vi "Main5.vi"(4 "מק\"ט המכלל":string, 5 "מספר סידורי":string, 7 "מפעיל":string="ANS", 8 "error":errorcluster, 11 "Path for Log":path) -> (0 "error IO":errorcluster)   [LabVIEW 2014]
uses:
  StopForLog.vi
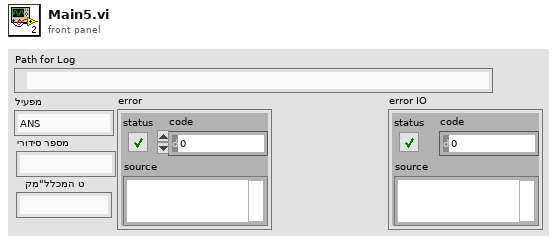
[diagram p1: front panel]
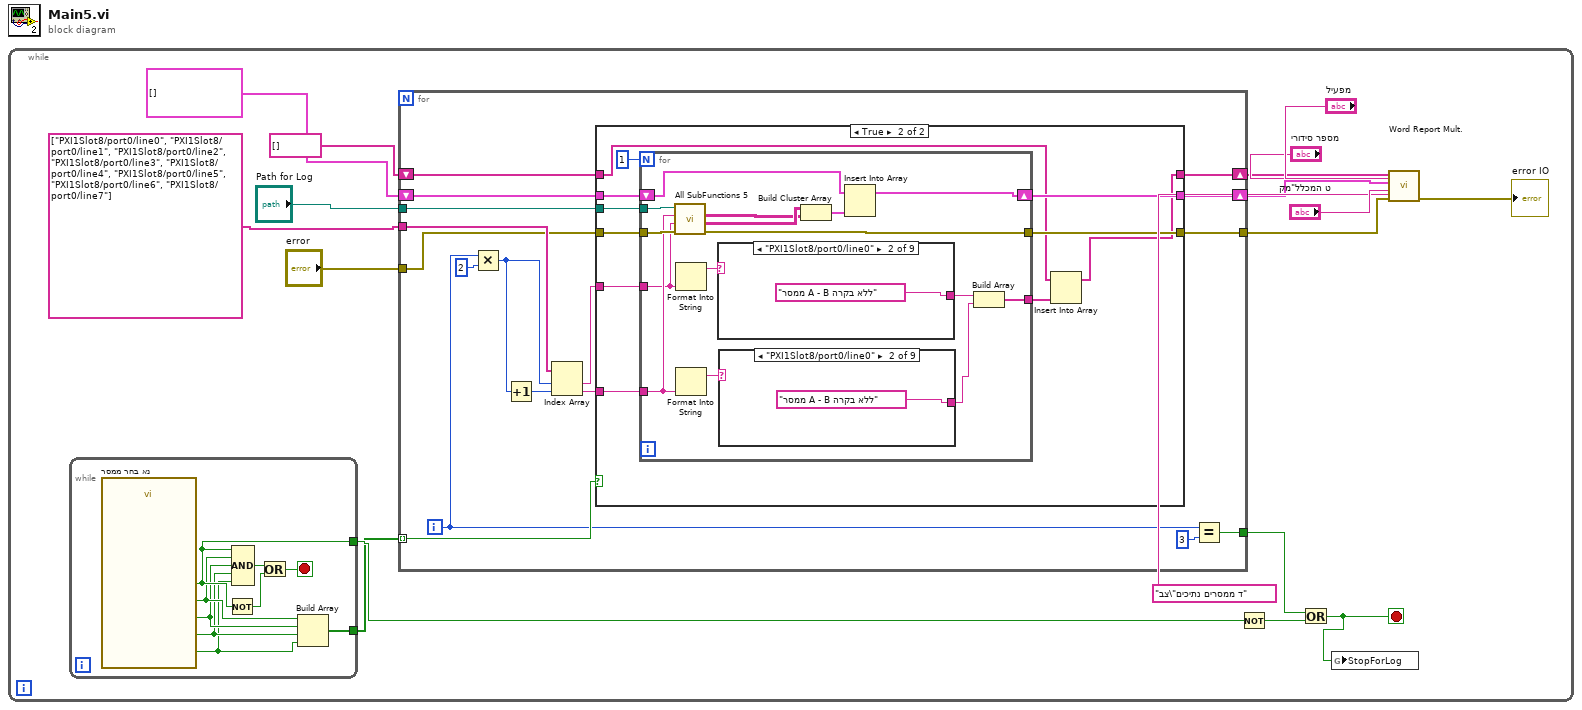
[diagram p0: block diagram]
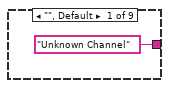
[diagram p3: hidden frame]
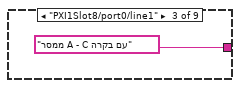
[diagram p4: hidden frame]
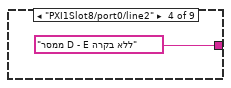
[diagram p5: hidden frame]
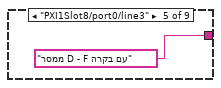
[diagram p6: hidden frame]
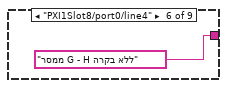
[diagram p7: hidden frame]
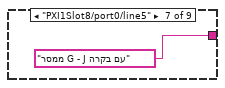
[diagram p8: hidden frame]
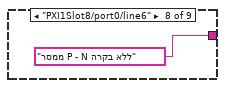
[diagram p9: hidden frame]
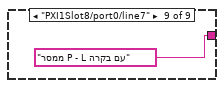
[diagram p10: hidden frame]
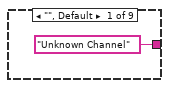
[diagram p11: hidden frame]
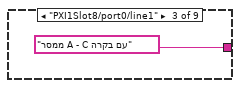
[diagram p12: hidden frame]
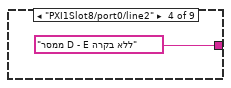
[diagram p13: hidden frame]
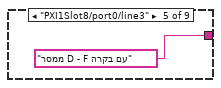
[diagram p14: hidden frame]
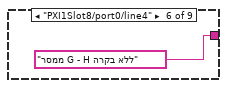
[diagram p15: hidden frame]
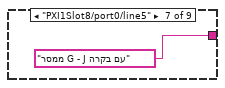
[diagram p16: hidden frame]
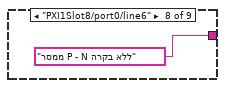
[diagram p17: hidden frame]
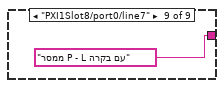
[diagram p18: hidden frame]
diagram:
  n1 = while {
    stop <- w1 stop-if-true
    n2 = while {
      tunnel: [w25] -> w18
      tunnel: [w26] -> w17
      stop <- w19 stop-if-true
      n3 = call "נא בחר ממסר.vi"() -> ("P - N/L"=w21:bool, "G - H/J"=w22:bool, "D - E/F"=w23:bool, "A - B/C"=w24:bool, "OK"=w25:bool)  [unwired: 13 in, 2 out]
      n4 = Not(x=w25) -> (.not. x?=w27:bool)
      n5 = Compound Arithmetic op=AND(w25, w24, w23, w22, w21) -> (w20:bool)
      n6 = Or(x=w20, y=w27) -> (x .or. y?=w19:bool)
      n7 = Build Array(w24, w23, w22, w21) -> (w26:bool[])
    }
    n8 = for {
      tunnel: w17 -> [w44] mode=indexing
      tunnel: tag[] ["PXI1Slot8/port0/line0", "PXI1Slot8/port0/line1", "PXI1Slot8/port0/line2", "PXI1Slot8/port0/line3", "PXI1Slot8/port0/line4", "PXI1Slot8/port0/line5", "PXI1Slot8/port0/line6", "PXI1Slot8/port0/line7"] -> [w43]
      tunnel: "Path for Log" -> [w37]
      tunnel: [w36] -> w6
      tunnel: "error" -> [w35]
      shift-right: [w33] -> w8
      shift-left: cluster{"appended array":string[][]}[] [] ("array of clusters") -> [w34]
      shift-right: [w31] -> w4
      shift-left: string[] [] ("Array 2") -> [w32]
      tunnel: [w28] -> w2
      i -> [w30]
      n9 = Multiply(x=w30, y=2) -> (x*y=w41:i32)
      n10 = Increment(x=w41) -> (x+1=w40:i32)
      n11 = Index Array(array=w43, index #1=w41, index #2=w40) -> (element #1=w39:tag, element #2=w38:tag)
      n12 = case shown="True" w44 {
        tunnel: w39 -> [_ w51]
        tunnel: w38 -> [_ w50]
        tunnel: w37 -> [_ w58]
        tunnel: [w47 w57] -> w36
        tunnel: w35 -> [w47 w56]
        tunnel: w34 -> [w46 w55]
        tunnel: [w46 w54] -> w33
        tunnel: w32 -> [w45 w53]
        tunnel: [w45 w52] -> w31
        frame False {
        }
        frame True {
          n13 = for {
            N: 1 -> [_]
            tunnel: w58 -> [w73]
            tunnel: [w72] -> w57
            tunnel: w56 -> [w71]
            shift-right: [w67] -> w54
            shift-left: w55 -> [w69]
            tunnel: w51 -> [w64]
            tunnel: w50 -> [w65]
            tunnel: [w66] -> w49
            n14 = call "All SubFunctions 5.vi"("error"=w71, "lines 1"=w64, "lines"=w65, "Path for Log"=w73) -> ("error IO"=w72:errorcluster, "appended array 1"=w62:string[][], "appended array"=w61:string[][])  [unwired: 5 in]
            n15 = Format Into String(w64) -> (resulting string=w70:string)  [unwired: 3 in, 1 out]
            n16 = Format Into String(w65) -> (resulting string=w59:string)  [unwired: 3 in, 1 out]
            n17 = case shown="\"PXI1Slot8/port0/line0\"" w70 {
              tunnel: ["Unknown Channel" "ממסר A - B ללא בקרה" "ממסר A - C עם בקרה" "ממסר D - E ללא בקרה" "ממסר D - F עם בקרה" "ממסר G - H ללא בקרה" "ממסר G - J עם בקרה" "ממסר P - N ללא בקרה" "ממסר P - L עם בקרה"] -> w63
              frame "", Default {
              }
              frame "PXI1Slot8/port0/line0" {
              }
              frame "PXI1Slot8/port0/line1" {
              }
              frame "PXI1Slot8/port0/line2" {
              }
              frame "PXI1Slot8/port0/line3" {
              }
              frame "PXI1Slot8/port0/line4" {
              }
              frame "PXI1Slot8/port0/line5" {
              }
              frame "PXI1Slot8/port0/line6" {
              }
              frame "PXI1Slot8/port0/line7" {
              }
            }
            n18 = case shown="\"PXI1Slot8/port0/line0\"" w59 {
              tunnel: ["Unknown Channel" "ממסר A - B ללא בקרה" "ממסר A - C עם בקרה" "ממסר D - E ללא בקרה" "ממסר D - F עם בקרה" "ממסר G - H ללא בקרה" "ממסר G - J עם בקרה" "ממסר P - N ללא בקרה" "ממסר P - L עם בקרה"] -> w60
              frame "", Default {
              }
              frame "PXI1Slot8/port0/line0" {
              }
              frame "PXI1Slot8/port0/line1" {
              }
              frame "PXI1Slot8/port0/line2" {
              }
              frame "PXI1Slot8/port0/line3" {
              }
              frame "PXI1Slot8/port0/line4" {
              }
              frame "PXI1Slot8/port0/line5" {
              }
              frame "PXI1Slot8/port0/line6" {
              }
              frame "PXI1Slot8/port0/line7" {
              }
            }
            n19 = Build Cluster Array(w62, w61) -> (w68:cluster{"appended array":string[][]}[])
            n20 = Insert Into Array(array=w69, new element=w68) -> (w67:cluster{"appended array":string[][]}[])  [unwired: 1 in]
            n21 = Build Array(w63, w60) -> (w66:string[])
          }
          n22 = Insert Into Array(array=w53, new element=w49) -> (w52:string[])  [unwired: 1 in]
        }
      }
      n23 = Equal?(x=w30, y=3) -> (x = y?=w28:bool)
    }
    n24 = Not(x=w18) -> (.not. x?=w3:bool)
    n25 = Or(x=w2, y=w3) -> (x .or. y?=w1:bool)
    n26 = global write "StopForLog.vi" "StopForLog"(w1) -> ()
    n27 = call "Word Report Mult..vi"("מפעיל"="מפעיל", "שם הצב\"ד"="צב\"ד ממסרים נתיכים", "מספר סידורי"="מספר סידורי", "error in (no error)"=w6, "מק\"ט המכלל"="מק\"ט המכלל", "Array of Items"=w8, "Elements"=w4) -> ("error out"=→"error IO":errorcluster)  [unwired: 4 in]
  }
